vi "Main1.2.vi"() -> ()   [LabVIEW 2017]
doc: "The myRIO Project template acquires acceleration data from the onboard accelerometer and displays the changes of acceleration values in a waveform chart."
uses:
  <vilib>/myRIO/Instrument Drivers/Onboard IO/DIO/typedefs/DIO Reference.ctl
  <vilib>/myRIO/Common/Instrument Driver Framework/Utilities/typedefs/myRIO Generic Hardware Reference.ctl
  <vilib>/myRIO/Common/Instrument Driver Framework/Utilities/typedefs/Hardware Version Enum.ctl
  <vilib>/myRIO/Common/Instrument Driver Framework/Utilities/typedefs/myRIO v1.0 Reference.ctl
  <vilib>/myRIO/Common/Instrument Driver Framework/Utilities/typedefs/Generic FPGA Reference.ctl
  <vilib>/myRIO/Common/Instrument Driver Framework/myRIO v1.0/DIO/typedefs/DIO Channels List.ctl
  <vilib>/myRIO/Common/Instrument Driver Framework/myRIO v1.0/DIO/typedefs/DIO Channels Enum.ctl
  <vilib>/userdefined/High Color/nirio_resource_hc.ctl
  <vilib>/myRIO/Common/Instrument Driver Framework/Utilities/vis/Is FPGA Ref Available.vi
  <vilib>/myRIO/Common/Instrument Driver Framework/myRIO v1.0/DIO/vis/myRIO v1.1 Open DIO.vi
  <vilib>/myRIO/Instrument Drivers/Onboard IO/DIO/vis/Write.vi
  <vilib>/myRIO/Common/Instrument Driver Framework/Utilities/vis/Validate Channels.vi
  <vilib>/myRIO/Common/Instrument Driver Framework/myRIO v1.0/DIO/vis/myRIO v1.0 Reserve DIO.vi
  <vilib>/myRIO/Common/Instrument Driver Framework/myRIO v1.0/UART/vis/myRIO v1.0 Close UART.vi
  <vilib>/myRIO/Common/Instrument Driver Framework/myRIO v1.0/Resource Manager/vis/myRIO v1.0 Reserve Channel List.vi
  <vilib>/myRIO/Common/Instrument Driver Framework/myRIO v1.0/DIO/vis/myRIO v1.0 Build MUX Configuration DIO.vi
  <vilib>/myRIO/Common/Instrument Driver Framework/myRIO v1.0/Resource Manager/vis/myRIO v1.0 Reserve Channel.vi
  <vilib>/myRIO/Common/Instrument Driver Framework/myRIO v1.0/Resource Manager/vis/myRIO v1.0 Unreserve Channel.vi
  <vilib>/myRIO/Common/Instrument Driver Framework/myRIO v1.0/Resource Manager/vis/myRIO v1.0 Create Configuration List.vi
  <vilib>/myRIO/Common/Instrument Driver Framework/myRIO v1.0/Resource Manager/vis/myRIO v1.0 Build Mutex Name.vi
  <vilib>/Utility/VariantDataType/GetNumericInfo.vi
  <vilib>/Utility/error.llb/Error Cluster From Error Code.vi
  <vilib>/myRIO/Common/Instrument Driver Framework/myRIO v1.0/myRIO v1.1 Open.vi
  <vilib>/myRIO/Common/Instrument Driver Framework/Utilities/vis/IO Manager.vi
  <vilib>/myRIO/Common/Instrument Driver Framework/Utilities/vis/Configuration Manager.vi
  <vilib>/myRIO/Common/Instrument Driver Framework/myRIO v1.0/Resource Manager/vis/myRIO v1.0 Configure IO.vi
  <vilib>/myRIO/Common/Instrument Driver Framework/myRIO v1.0/myRIO v1.0 Close.vi
  <vilib>/myRIO/Common/Instrument Driver Framework/myRIO v1.0/DIO/vis/myRIO v1.0 Write DIO.vi
  Globales.vi
  <vilib>/myRIO/Common/Instrument Driver Framework/Utilities/vis/FPGA Ref Manager.vi
  <vilib>/myRIO/Common/Instrument Driver Framework/myRIO v1.0/myRIO v1.0 Reset FPGA.vi
  <vilib>/myRIO/Common/Instrument Driver Framework/myRIO v1.0/IRQ/vis/myRIO v1.0 IRQ Info FGV.vi
  <vilib>/myRIO/Common/Instrument Driver Framework/myRIO v1.0/IRQ/vis/myRIO v1.0 Timer IRQ Info FGV.vi
  <vilib>/myRIO/Common/Instrument Driver Framework/myRIO v1.0/IRQ/vis/myRIO v1.0 ISR Agent.vi
  <vilib>/myRIO/Express VI/Onboard IO/DO/DO Express VI.xnode
  <vilib>/myRIO/Instrument Drivers/Onboard IO/DIO/vis/myRIO DIO Open.xnode
  <vilib>/myRIO/Instrument Drivers/Utilities/Utilities.lvlib
  <vilib>/myRIO/Instrument Drivers/Onboard IO/DIO/DIO.lvlib
panel:
  in  "Calibrar":bool
  in  "Home":bool
  in  "Ir_posicion":bool
  in  "Fijar Posición":dbl
  out "Posición en X":dbl
  in  "Arriba_X":bool
  in  "Abajo_X":bool
  in  "Avance":dbl
  out "error out":errorcluster
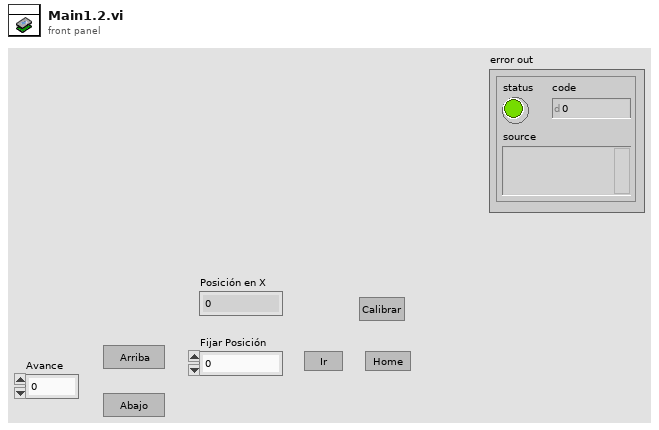
[diagram p1: front panel]
types:
  T1 = typedef "DIO.lvlib/DIO Reference.ctl" = cluster{"myRIO Reference":T2, "DIO Channels List":T6}
  T2 = typedef "myRIO Generic Hardware Reference.ctl" = cluster{"myRIO Model":T3, "myRIO Hardware Reference":T4}
  T3 = typedef "Hardware Version Enum.ctl" = enum16{"Unknown", "myRIO-1900", "myRIO-1950", "roboRIO", "NI ELVIS RIO CM"}
  T4 = typedef "myRIO v1.0 Reference.ctl" = cluster{"Generic FPGA Reference":T5, "Allow multiple opens":bool}
  T5 = typedef "Generic FPGA Reference.ctl" = refnum<k20>
  T6 = typedef "DIO Channels List.ctl" = T7[]
  T7 = typedef "DIO Channels Enum.ctl" = enum16{"Not Connected", "C/DIO0", "C/DIO1", "C/DIO2", "C/DIO3", "C/DIO4", "C/DIO5", "C/DIO6", "C/DIO7", "A/DIO0", "A/DIO1", "A/DIO2", "A/DIO3", "A/DIO4", "A/DIO5", "A/DIO6", "A/DIO7", "A/DIO8", "A/DIO9", "A/DIO10", "A/DIO11", "A/DIO12", "A/DIO13", "A/DIO14", "A/DIO15", "B/DIO0", "B/DIO1", "B/DIO2", "B/DIO3", "B/DIO4", "B/DIO5", "B/DIO6", "B/DIO7", "B/DIO8", "B/DIO9", "B/DIO10", "B/DIO11", "B/DIO12", "B/DIO13", "B/DIO14", "B/DIO15", "LED0", "LED1", "LED2", "LED3", "Button0", "DIO/DIO0", "DIO/DIO1", "DIO/DIO2", "DIO/DIO3", "DIO/DIO4", "DIO/DIO5", "DIO/DIO6", "DIO/DIO7", "DIO/DIO8", "DIO/DIO9", "SPI/CS0", "SPI/CS1", "SPI/CS2", "SPI/CS3", "LED RADIO (Green)", "LED RADIO (Red)", "LED COMM (Green)", "LED COMM (Red)", "LED MODE (Green)", "LED MODE (Red)"}
  T8 = typedef "nirio_resource_hc.ctl" = tag
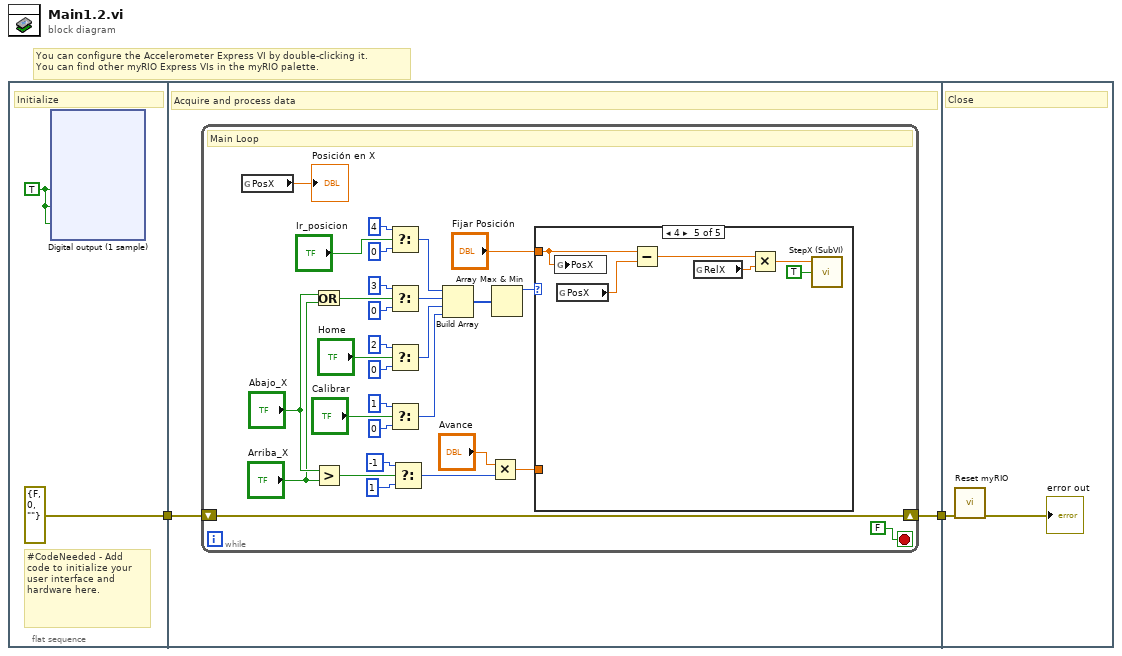
[diagram p0: block diagram]
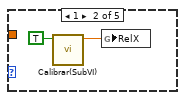
[diagram p3: hidden frame]
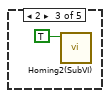
[diagram p4: hidden frame]
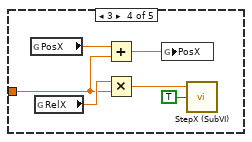
[diagram p5: hidden frame]
diagram:
  # "You can configure the Accelerometer Express VI by double-clicking it.\nYou can find other myRIO Express VIs in the myRIO palette."
  n1 = flat-sequence {
    tunnel: [errorcluster {"status"=FALSE, "code"=0, "source"=""} ("error in (no error)")] -> w2
    tunnel: w2 -> [w43]
    tunnel: [w42] -> w1
    tunnel: w1 -> [w90]
    frame #0 {
      w3 = TRUE
      # "#CodeNeeded - Add code to initialize your user interface and hardware here."
      # "Initialize"
      n2 = xnode "Digital output (1 sample)"("Direccion (A/DIO0 (Pin 11))"=w3, "Step (A/DIO1 (Pin 13))"=w3, "ON/OFF (A/DIO4 (Pin 19))"=w3) -> ()  [unwired: 1 in, 1 out]
    }
    frame #1 {
      # "Acquire and process data"
      n3 = while {
        shift-right: [w47] -> w42
        shift-left: w43 -> [w47]
        stop <- FALSE stop-if-true
        # "Main Loop"
        n4 = global read "Globales.vi" "PosX"() -> (→"Posición en X":dbl)
        n5 = Or(x="Abajo_X", y="Arriba_X") -> (x .or. y?=w63:bool)
        n6 = Greater?(x="Abajo_X", y="Arriba_X") -> (0:w53:bool)
        n7 = Select(t=4, s="Ir_posicion", f=0) -> (s? t:f=w61:i32)
        n8 = Select(t=3, s=w63, f=0) -> (s? t:f=w60:i32)
        n9 = Select(t=2, s="Home", f=0) -> (s? t:f=w59:i32)
        n10 = Select(t=1, s="Calibrar", f=0) -> (s? t:f=w58:i32)
        n11 = Select(t=-1, s=w53, f=1) -> (s? t:f=w49:i32)
        n12 = Build Array(w61, w60, w59, w58) -> (w57:i32[])
        n13 = Multiply(x="Avance", y=w49) -> (x*y=w45:dbl)
        n14 = Array Max & Min(array=w57) -> (max value=w56:i32)  [unwired: 3 out]
        n15 = case shown="4" w56 {
          tunnel: w45 -> [_ _ _ w79 _]
          tunnel: "Fijar Posición" -> [_ _ _ _ w85]
          frame 0, Default {
          }
          frame 1 {
            n16 = call "Calibrar(SubVI).vi"("Calibrar"=TRUE) -> ("Relación"=w74:dbl)  [unwired: 10 in]
            n17 = global write "Globales.vi" "RelX"(w74) -> ()
          }
          frame 2 {
            n18 = call "Homing2(SubVI).vi"("Home"=TRUE) -> ()  [unwired: 10 in, 1 out]
          }
          frame 3 {
            n19 = global read "Globales.vi" "PosX"() -> (w80:dbl)
            n20 = global read "Globales.vi" "RelX"() -> (w82:dbl)
            n21 = Add(x=w80, y=w79) -> (x+y=w81:dbl)
            n22 = Multiply(x=w82, y=w79) -> (x*y=w78:dbl)
            n23 = global write "Globales.vi" "PosX"(w81) -> ()
            n24 = call "StepX (SubVI).vi"("Mover"=TRUE, "Step"=w78) -> ()  [unwired: 3 in]
          }
          frame 4 {
            n25 = global write "Globales.vi" "PosX"(w85) -> ()
            n26 = global read "Globales.vi" "PosX"() -> (w88:dbl)
            n27 = Subtract(x=w85, y=w88) -> (x-y=w87:dbl)
            n28 = global read "Globales.vi" "RelX"() -> (w86:dbl)
            n29 = Multiply(x=w87, y=w86) -> (x*y=w83:dbl)
            n30 = call "StepX (SubVI).vi"("Mover"=TRUE, "Step"=w83) -> ()  [unwired: 3 in]
          }
        }
      }
    }
    frame #2 {
      # "Close"
      n31 = call <vilib>:"Reset myRIO.vi"("error in (no error)"=w90) -> ("error out"=→"error out":errorcluster)  [unwired: 10 in]
    }
  }
